vi "Commutator_init.vi"(3 "VISA resource name":refnum<visa-resource-name>) -> (0 "status":bool, 1 "VISA out":T1)   [LabVIEW 2017]
uses:
  <vilib>/Instr/_visa.llb/VISA Configure Serial Port (Instr).vi
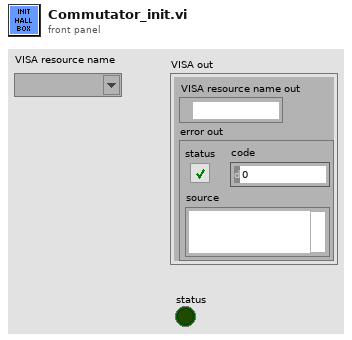
[diagram p1: front panel]
types:
  T1 = cluster{"VISA resource name out":refnum<visa-resource-name>, "error out":errorcluster}
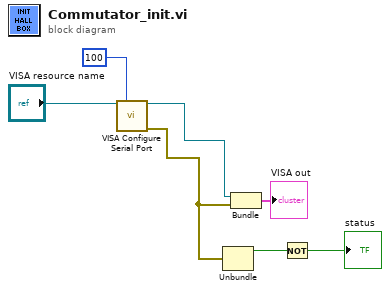
[diagram p0: block diagram]
diagram:
  n1 = call-poly "VISA Configure Serial Port"("VISA resource name"="VISA resource name", "timeout (10sec)"=u32 100) -> ("VISA resource name out"=w5:refnum<visa-resource-name>, "error out"=w3:errorcluster)  [unwired: 12 in]
  n2 = Unbundle(w3) -> ("status"=w1:bool)  [unwired: 2 out]
  n3 = Bundle("VISA resource name out"=w5, "error out"=w3) -> (→"VISA out":T1)  [unwired: 1 in]
  n4 = Not(x=w1) -> (.not. x?=→"status":bool)
